vi "AIT 664 - Parse Sysdef.vi"(0 "Device Reference in":T3 format="%.0x", 5 "End System Handle in":u64 format="%x", 7 "FIFO Index Queues":T2, 11 "error in (no error)":errorcluster) -> (4 "Hardware Input - Rx Section Data":T4[](array[typedef]) {"Message Settings"."Transmit Channel Data Reference" format="%.0x"; "Message Settings"."Queue Transmit Channel" format="%.0x"; "Message Settings"."Driver Data"."Num Bits" min=1 max=32; "Message Settings"."Block Data Refs"."Data Reference" format="%.0x"; "Rx Com Udp Port"."Handle" format="%08x"; "Tx Com Udp Port"."Handle" format="%08x"}, 6 "Hardware Output - Tx Section Data":T4[](array[typedef]) {"Message Settings"."Transmit Channel Data Reference" format="%.0x"; "Message Settings"."Queue Transmit Channel" format="%.0x"; "Message Settings"."Driver Data"."Num Bits" min=1 max=32; "Message Settings"."Block Data Refs"."Data Reference" format="%.0x"; "Rx Com Udp Port"."Handle" format="%08x"; "Tx Com Udp Port"."Handle" format="%08x"}, 8 "output cluster":T1, 15 "error out":errorcluster)   [LabVIEW 2013, in "AIT 664 Custom Device.lvlib"]
doc: "Build the Hardware Input Rx, and Hardware Output Tx channel data.\n\nReturns built Hardware Input Rx and Hardware Output Tx channel data and the buffer indicies and buffer lengths for each hardware channel, in and out."
uses:
  AIT 664 Custom Device.lvlib
  RT Controls/AIT 664 - RT Hardware Channel.ctl
  RT Controls/AIT 664 - RT Message Settings.ctl
  <vilib>/NI Veristand/Custom Device API/Block Data Reference.ctl
  <vilib>/NI Veristand/Custom Device API/Data Reference.ctl
  RT Controls/AIT 664 - Driver Data.ctl
  Controls and Global/Start Bit.ctl
  Controls and Global/Number of Bits.ctl
  <vilib>/NI Veristand/Custom Device API/Custom Device Item Ref.ctl
  <userlib>/ARINC 664/AIT 664 Controls/General/Message Port.ctl
  <userlib>/ARINC 664/AIT 664 Controls/General/Direction.ctl
  <userlib>/ARINC 664/AIT 664 Controls/General/Message Port Type.ctl
  System Explorer/Controls/664 - Sampling Type.ctl
  RT Controls/FIFO Index Queues.ctl
  RT Controls/FIFO.ctl
  <vilib>/NI Veristand/Custom Device Tools/Custom Device Utility Library/Custom Device Utility Library.lvlib
  <vilib>/NI Veristand/Custom Device API/Custom Device API.lvlib
  <userlib>/ARINC 664/AIT 664 API.lvlib
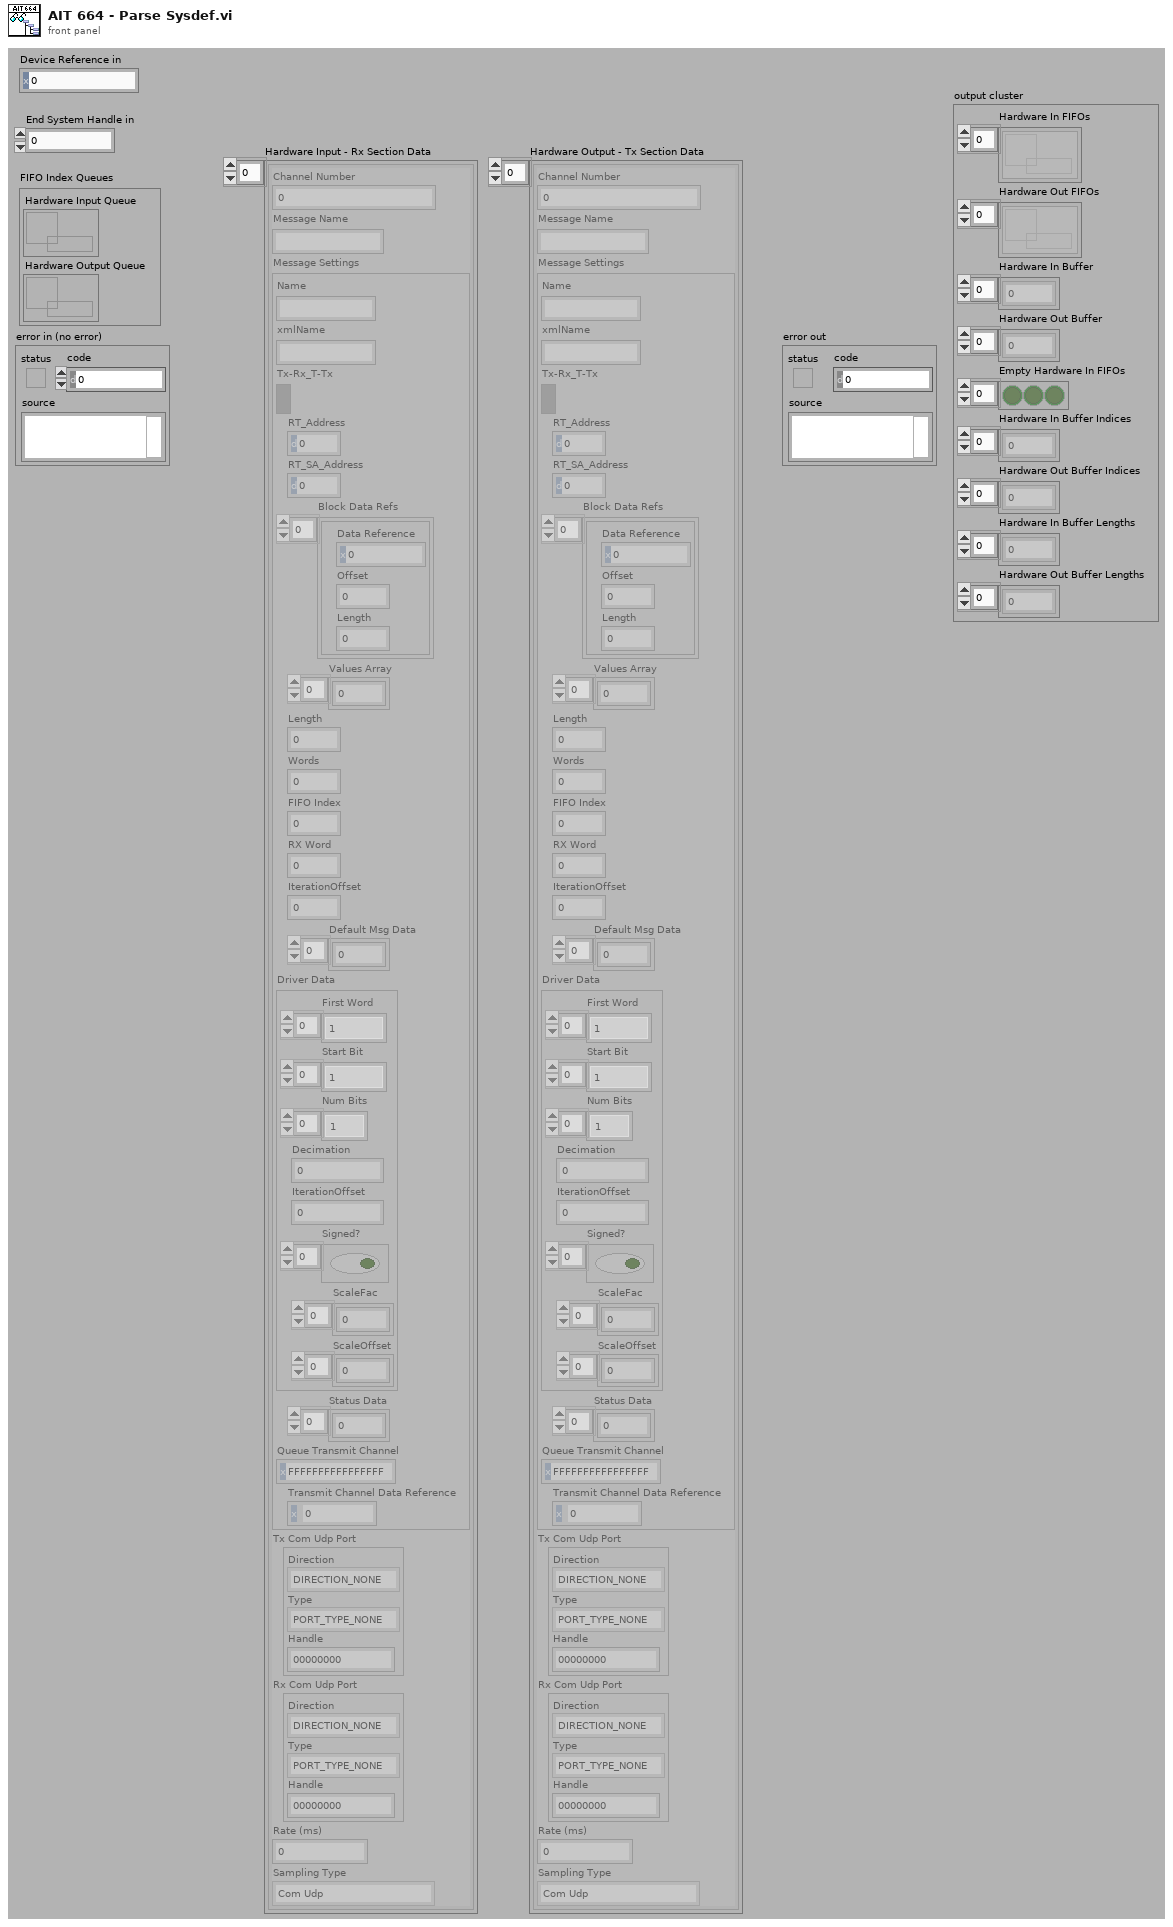
[diagram p1: front panel]
types:
  T1 = typedef "AIT 664 Custom Device.lvlib/FIFO.ctl" = cluster{"Hardware In FIFOs":refnum<k33>[], "Hardware Out FIFOs":refnum<k33>[], "Hardware In Buffer":dbl[], "Hardware Out Buffer":dbl[], "Empty Hardware In FIFOs":bool[], "Hardware In Buffer Indices":i32[], "Hardware Out Buffer Indices":i32[], "Hardware In Buffer Lengths":i32[], "Hardware Out Buffer Lengths":i32[]}
  T2 = typedef "AIT 664 Custom Device.lvlib/FIFO Index Queues.ctl" = cluster{"Hardware Input Queue":refnum<queue>, "Hardware Output Queue":refnum<queue>}
  T3 = typedef "Custom Device API.lvlib/Custom Device Item Ref.ctl" = u64
  T4 = typedef "AIT 664 Custom Device.lvlib/AIT 664 - RT Hardware Channel.ctl" = cluster{"Channel Number":u16, "Message Name":string, "Message Settings":T5, "Tx Com Udp Port":T11, "Rx Com Udp Port":T11, "Rate (ms)":u32, "Sampling Type":T14}
  T5 = typedef "AIT 664 Custom Device.lvlib/AIT 664 - RT Message Settings.ctl" = cluster{"Name":string, "xmlName":string, "Tx-Rx_T-Tx":bool, "RT_Address":u8, "RT_SA_Address":u8, "Block Data Refs":T6[], "Values Array":dbl[], "Length":i32, "Words":i32, "FIFO Index":i32, "RX Word":u32, "IterationOffset":i32, "Default Msg Data":u8[], "Driver Data":T8, "Status Data":u32[], "Queue Transmit Channel":T3, "Transmit Channel Data Reference":T7}
  T6 = typedef "Custom Device API.lvlib/Block Data Reference.ctl" = cluster{"Data Reference":T7, "Offset":i32, "Length":i32}
  T7 = typedef "Custom Device API.lvlib/Data Reference.ctl" = i32
  T8 = typedef "AIT 664 Custom Device.lvlib/AIT 664 - Driver Data.ctl" = cluster{"First Word":T9[], "Start Bit":T9[], "Num Bits":T10[], "Decimation":i32, "IterationOffset":i32, "Signed?":bool[], "ScaleFac":dbl[], "ScaleOffset":dbl[]}
  T9 = typedef "AIT 664 Custom Device.lvlib/Start Bit.ctl" = i32
  T10 = typedef "AIT 664 Custom Device.lvlib/Number of Bits.ctl" = i32
  T11 = typedef "AIT 664 API.lvlib/Message Port.ctl" = cluster{"Direction":T12, "Type":T13, "Handle":u64}
  T12 = typedef "AIT 664 API.lvlib/Direction.ctl" = enum16{"DIRECTION_NONE", "DIRECTION_TX", "DIRECTION_RX"}
  T13 = typedef "AIT 664 API.lvlib/Message Port Type.ctl" = enum16{"PORT_TYPE_NONE", "COM_UDP", "SAP_UDP", "SAP_IP", "SAP_MAC", "COTS_MAC", "COTS_MAC_RAW"}
  T14 = typedef "AIT 664 Custom Device.lvlib/664 - Sampling Type.ctl" = enum16{"Com Udp", "Com Udp Queuing", "Sap Udp", "Sap Ip", "Sap Mac", "Unknown"}
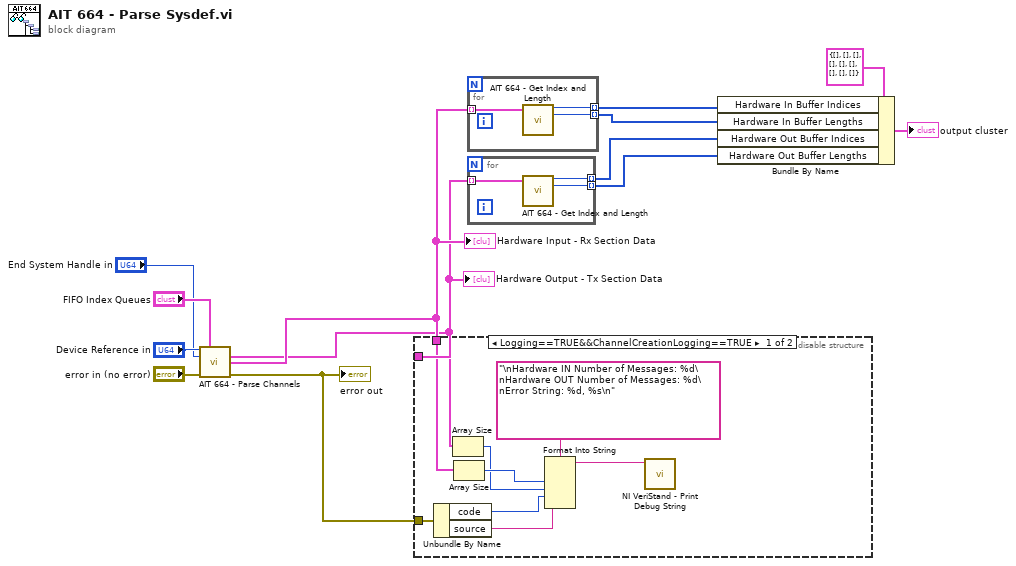
[diagram p0: block diagram]
diagram:
  n1 = call "AIT 664 - Parse Channels.vi"("Device Reference in"="Device Reference in", "FIFO Index Queues"="FIFO Index Queues", "End System Handle in"="End System Handle in", "error in (no error)"="error in (no error)") -> ("Hardware Output - Tx Ports"=w1:T4[], "Hardware Input  -Rx Ports"=w2:T4[], "error out"=w3:errorcluster)  [unwired: 9 in]
  "Hardware Output - Tx Section Data" <- w1
  "Hardware Input - Rx Section Data" <- w2
  "error out" <- w3
  n2 = disable-structure shown="Logging==TRUE&&ChannelCreationLogging==TRUE" {
    disable-tunnel: w2 -> [w17 _]
    disable-tunnel: w1 -> [w16 _]
    disable-tunnel: w3 -> [w15 _]
    frame condition #0 (active) {
      n3 = Unbundle By Name(w15) -> ("code"=w19:i32, "source"=w18:string)
      n4 = Array Size(array=w16) -> (size(s)=w20:i32)
      n5 = Array Size(array=w17) -> (size(s)=w21:i32)
      n6 = Format Into String(format string="\nHardware IN Number of Messages: %d\nHardware OUT Number of Messages: %d\nError String: %d, %s\n", w21, w20, w19, w18) -> (resulting string=w14:string)  [unwired: 2 in, 1 out]
      n7 = call <vilib>:"NI VeriStand - Print Debug String.vi"("Message"=w14) -> ()  [unwired: 10 in, 1 out]
    }
    frame condition #1 {
    }
  }
  n8 = for {
    tunnel: w2 -> [w25] mode=indexing
    tunnel: [w24] -> w9 mode=indexing
    tunnel: [w23] -> w8 mode=indexing
    n9 = call "AIT 664 - Get Index and Length.vi"("Section"=w25) -> ("FIFO Index"=w24:i32, "Length"=w23:i32)  [unwired: 13 in]
  }
  n10 = for {
    tunnel: w1 -> [w28] mode=indexing
    tunnel: [w27] -> w7 mode=indexing
    tunnel: [w26] -> w6 mode=indexing
    n11 = call "AIT 664 - Get Index and Length.vi"("Section"=w28) -> ("FIFO Index"=w27:i32, "Length"=w26:i32)  [unwired: 13 in]
  }
  n12 = Bundle By Name(cluster=T1 {"Hardware In FIFOs"=[], "Hardware Out FIFOs"=[], "Hardware In Buffer"=[], "Hardware Out Buffer"=[], "Empty Hardware In FIFOs"=[], "Hardware In Buffer Indices"=[], "Hardware Out Buffer Indices"=[], "Hardware In Buffer Lengths"=[], "Hardware Out Buffer Lengths"=[]} ("output cluster"), "Hardware In Buffer Indices"=w9, "Hardware In Buffer Lengths"=w8, "Hardware Out Buffer Indices"=w7, "Hardware Out Buffer Lengths"=w6) -> (→"output cluster":T1)
